vi "QNET_ROTPEN_Enable_Balance.vi"(2 "Previous State":bool, 3 "alpha_dot (rad/s)":dbl, 4 "alpha_up (rad)":dbl) -> (0 "Current State":bool, 1 "In Range?":bool)   [LabVIEW 2021]
doc: "This VI determines when the balance controller should be activated. The pendulum is in range if all of these are true:\n(1) Angular speed is within +/- 720 deg/s\n(2) Pendulum within +/- 30 deg of vertical.\n(3) Pendulum is within +/- 2 deg of the vertical OR was within +/- 2 deg of vertical in the previous sample."
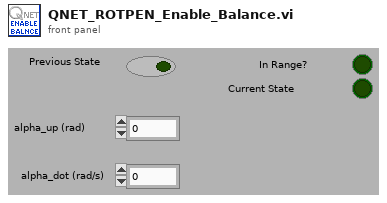
[diagram p1: front panel]
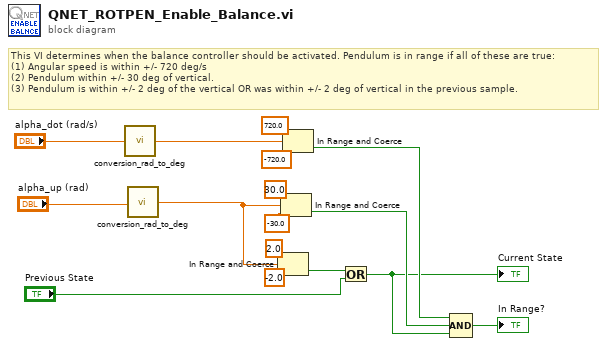
[diagram p0: block diagram]
diagram:
  # "This VI determines when the balance controller should be activated. Pendulum is in range if all of these are true:\n(1) Angular speed is within +/- 720 deg/s\n(2) Pendulum within +/- 30 deg of vertical.\n(3) Pendulum is within +/- 2 deg of the vertical OR was within +/- 2 deg of vertical in the previous sample."
  n1 = call "conversion_rad_to_deg.vi"("Angle (rad)"="alpha_dot (rad/s)") -> ("Angle (deg)"=w3:dbl)
  n2 = call "conversion_rad_to_deg.vi"("Angle (rad)"="alpha_up (rad)") -> ("Angle (deg)"=w1:dbl)
  n3 = In Range and Coerce(upper limit=sgl 2.0, x=w1, lower limit=sgl -2.0) -> (In Range?=w12:bool)  [unwired: 1 out]
  n4 = In Range and Coerce(upper limit=sgl 30.0, x=w1, lower limit=sgl -30.0) -> (In Range?=w7:bool)  [unwired: 1 out]
  n5 = In Range and Coerce(upper limit=sgl 720.0, x=w3, lower limit=sgl -720.0) -> (In Range?=w8:bool)  [unwired: 1 out]
  n6 = Or(x=w12, y="Previous State") -> (x .or. y?=w6:bool)
  "Current State" <- w6
  n7 = Compound Arithmetic op=AND(w8, w7, w6) -> (→"In Range?":bool)
